vi "Remove_Duplicate_Chs.vi"(0 "Filename":path, 11 "Start of read offset (chars.: 0)":i32) -> ()   [LabVIEW 2010]
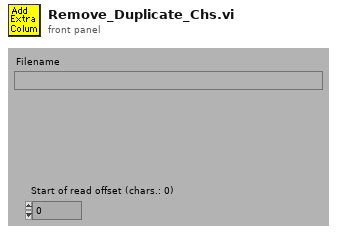
[diagram p1: front panel]
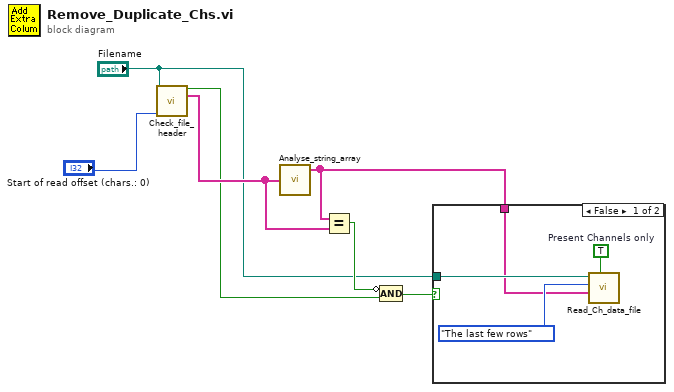
[diagram p0: block diagram]
diagram:
  n1 = call "Check_file_header.vi"("Filename"="Filename", "Start of read offset (chars.: 0)"="Start of read offset (chars.: 0)") -> ("exists?"=w3:bool, "Merged Channels"=w5:string[])  [unwired: 7 in, 5 out]
  n2 = call "Analyse_string_array.vi"("String array"=w5) -> ("Unique strings"=w6:string[])  [unwired: 1 in, 1 out]
  n3 = Equal?(x=w6, y=w5) -> (x = y?=w4:bool)
  n4 = Compound Arithmetic op=AND(invert w4, w3) -> (w2:bool)
  n5 = case shown="False" w2 {
    tunnel: "Filename" -> [w11 _]
    tunnel: w6 -> [w8 _]
    frame False {
      w9 = TRUE  # Present Channels only
      n6 = call "Read_Ch_data_file.vi"("Present Channels only"=w9, "Present Channels"=w8, "Output"=enum16{"All Ch data", "The last few rows"}."The last few rows", "Filename"=w11) -> ()  [unwired: 1 in, 5 out]
    }
    frame True {
    }
  }
